vi "Convert Modifiers to String.vi"(9 "Shift?":bool, 10 "Alt?":bool, 11 "Ctrl?":bool) -> (3 "String":string)   [LabVIEW 2020, in "MacroAssert.lvlib"]
doc: "Converts the modifiers to a string to be displayed."
uses:
  MacroAssert.lvlib
  <userlib>/_OpenG.lib/array/array.llb/Filter 1D Array with Scalar (String)__ogtk.vi
  <userlib>/_OpenG.lib/array/array.llb/openg_array.lvlib
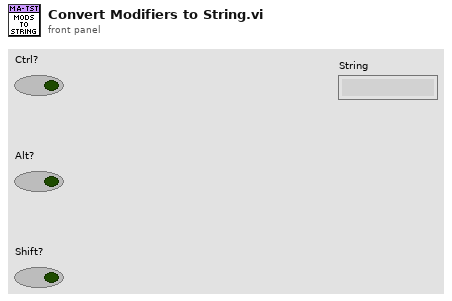
[diagram p1: front panel]
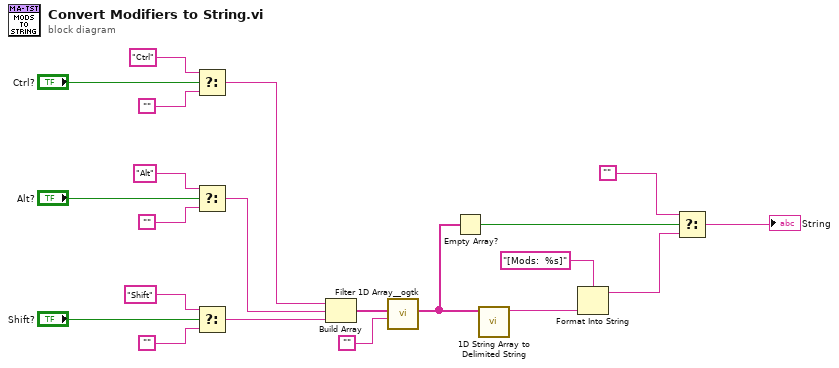
[diagram p0: block diagram]
diagram:
  n1 = Select(t="Ctrl", s="Ctrl?", f="") -> (s? t:f=w12:string)
  n2 = Select(t="Alt", s="Alt?", f="") -> (s? t:f=w11:string)
  n3 = Select(t="Shift", s="Shift?", f="") -> (s? t:f=w10:string)
  n4 = Build Array(w12, w11, w10) -> (w9:string[])
  n5 = call-poly <userlib>:"Filter 1D Array__ogtk.vi"("items to filter"="", "array"=w9) -> ("filtered array"=w7:string[])  [unwired: 4 in, 1 out]
  n6 = Empty Array?(array=w7) -> (empty?=w4:bool)
  n7 = call <vilib>:"1D String Array to Delimited String.vi"("string array"=w7) -> ("delimited string"=w5:string)  [unwired: 10 in]
  n8 = Format Into String(format string="[Mods:  %s]", w5) -> (resulting string=w3:string)  [unwired: 2 in, 1 out]
  n9 = Select(t="", s=w4, f=w3) -> (s? t:f=→"String":string)
